vi "File Analysis Tools.vi"() -> ()   [LabVIEW 2024]
panel:
  out "appended array":string[][](array[string])
  in  "Analyze Button":bool
  out "the file matches a signature":string
  out "the file matches a signature":bool
  out "Hex Viewer Table":string[][](table)
  in  "File Metadata Table":string[][](table)
  in  "Path":path
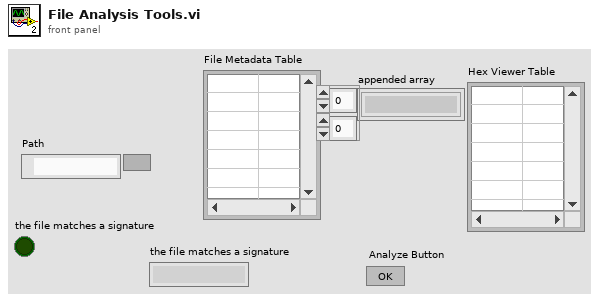
[diagram p1: front panel]
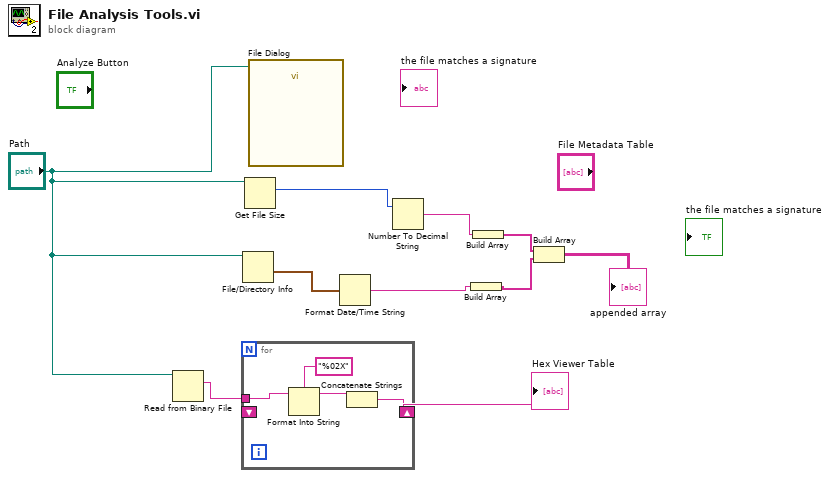
[diagram p0: block diagram]
diagram:
  n1 = Read from Binary File(11:"Path") -> (2:w2:string)  [unwired: 5 in, 3 out]
  n2 = for {
    tunnel: w2 -> [w13]
    shift-right: [w11] -> w1
    shift-left: _ -> [_]
    n3 = Format Into String(format string="%02X", initial string=w13) -> (resulting string=w12:string)  [unwired: 2 in, 1 out]
    n4 = Concatenate Strings(w12) -> (w11:string)  [unwired: 1 in]
  }
  "Hex Viewer Table" <- w1
  n5 = File/Directory Info(path="Path") -> (last mod=w10:timestamp)  [unwired: 1 in, 6 out]
  n6 = Get File Size(file="Path") -> (size (in bytes)=w9:i64)  [unwired: 1 in, 2 out]
  n7 = call "File Dialog"("start path"="Path") -> ()  [unwired: 11 in, 4 out]
  n8 = Format Date/Time String(seconds (now)=w10) -> (date/time string=w7:string)  [unwired: 2 in]
  n9 = Number To Decimal String(number=w9) -> (decimal integer string=w8:string)  [unwired: 1 in]
  n10 = Build Array(w7) -> (w5:string[])
  n11 = Build Array(w8) -> (w6:string[])
  n12 = Build Array(w6, w5) -> (→"appended array":string[][])
